vi "StationInfo@StateShift__Parameter.vi"(1 "ParamterIn":string) -> (0 "ParamterOut":string)   [LabVIEW 2020]
panel:
  in  "Offset":string(combo)
  in  "Confirm":bool
  # "StationInfo@StateShift $Offset"
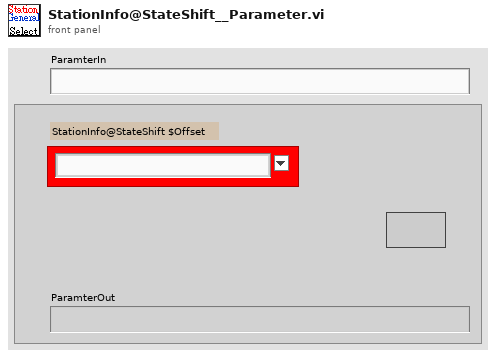
[diagram p1: front panel]
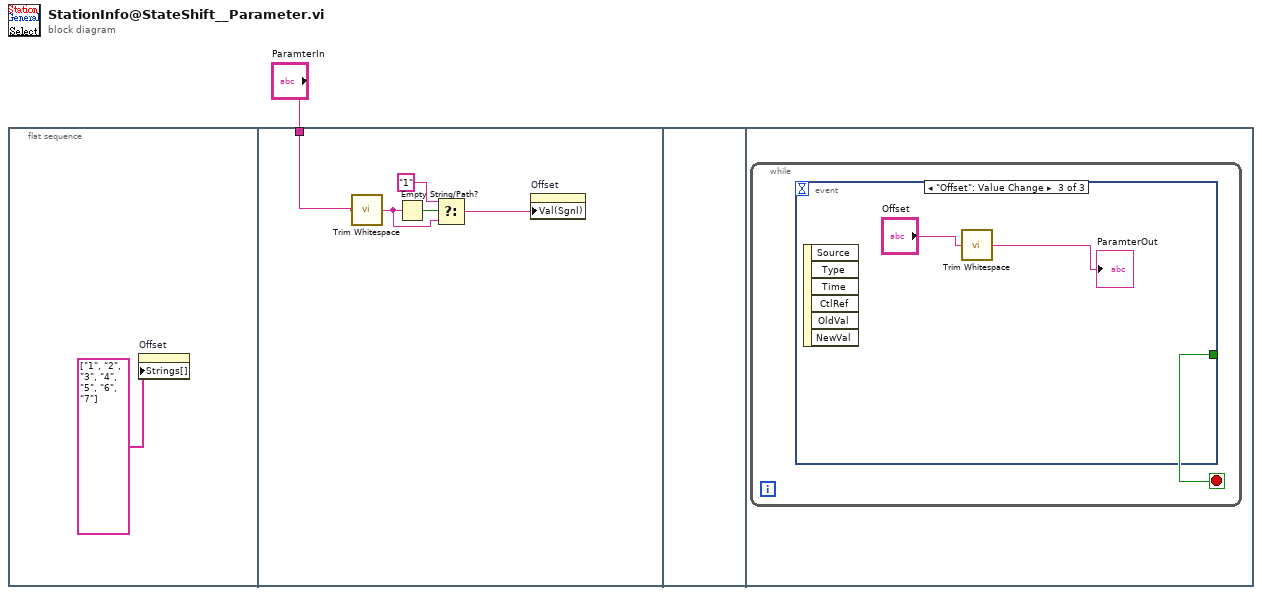
[diagram p0: block diagram]
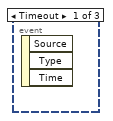
[diagram p2: hidden frame]
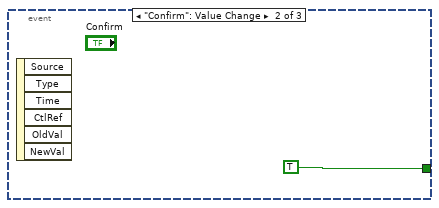
[diagram p3: hidden frame]
diagram:
  n1 = flat-sequence {
    tunnel: "ParamterIn" -> [w7]
    frame #0 {
      n2 = property on="Offset" class="CmbBox"("Strings[]"=string[] ["1", "2", "3", "4", "5", "6", "7"] ("Strings []")) -> ()  [unwired: 2 in, 2 out]
    }
    frame #1 {
      n3 = call <vilib>:"Trim Whitespace.vi"("string"=w7) -> ("trimmed string"=w5:string)  [unwired: 1 in]
      n4 = Empty String/Path?(string/path=w5) -> (empty?=w6:bool)
      n5 = Select(t="1", s=w6, f=w5) -> (s? t:f=w3:string)
      n6 = property on="Offset" class="CmbBox"("Val(Sgnl)"=w3) -> ()  [unwired: 2 in, 2 out]
    }
    frame #2 {
    }
    frame #3 {
      n7 = while {
        stop <- w8 stop-if-true
        n8 = event shown="[2] \"Offset\": Value Change" {
          selector: _ -> [_ _ _]
          dyn-events: _ -> [_ _ _]
          timeout: _ -> [_ _ _]
          tunnel: [_ TRUE _] -> w8
          event Timeout {
            n9 = event-data() -> ()  [unwired: 1 in, 3 out]
          }
          event "Confirm": Value Change {
            n10 = event-data() -> ()  [unwired: 1 in, 6 out]
          }
          event "Offset": Value Change {
            n11 = event-data() -> ()  [unwired: 1 in, 6 out]
            n12 = call <vilib>:"Trim Whitespace.vi"("string"="Offset") -> ("trimmed string"=→"ParamterOut":string)  [unwired: 1 in]
          }
        }
      }
    }
  }
